vi "SetSystemDefinitionPropertyValue.vi"(8 "error in (no error)":errorcluster, 9 "value":string, 10 "property name":string, 11 "BaseNodeType in":refnum<k24>) -> (0 "error out":errorcluster, 3 "BaseNodeType out":refnum<k24>)   [LabVIEW 2015, in "VeriStandTestUtilities.lvlib"]
uses:
  VeriStandTestUtilities.lvlib
  NationalInstruments.VeriStand.SystemStorage
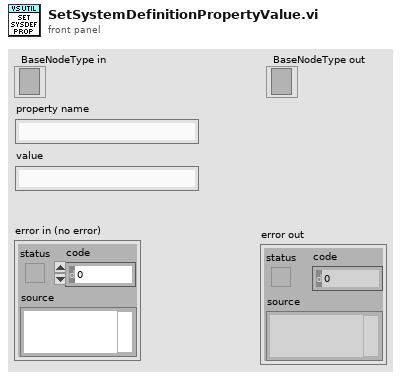
[diagram p1: front panel]
types:
  T1 = typedef "PropertyType.ctl" = enum16{"K_STRING", "K_BOOL", "K_I32", "K_U32", "K_DOUBLE", "K_U64", "K_VARIANT", "K_DEPENDENTFILE", "K_DEPENDENTNODE", "K_DATASOURCENODE", "K_U16", "K_DBLARR", "K_U32ARR", "K_I32ARR", "K_STRINGARR", "K_DICTIONARY", "K_DICTIONARYARR", "K_BINARYSTRING", "K_I16", "K_I64", "K_BOOLARR", "K_U64ARR", "K_U16ARR", "K_I64ARR", "K_I16ARR"}
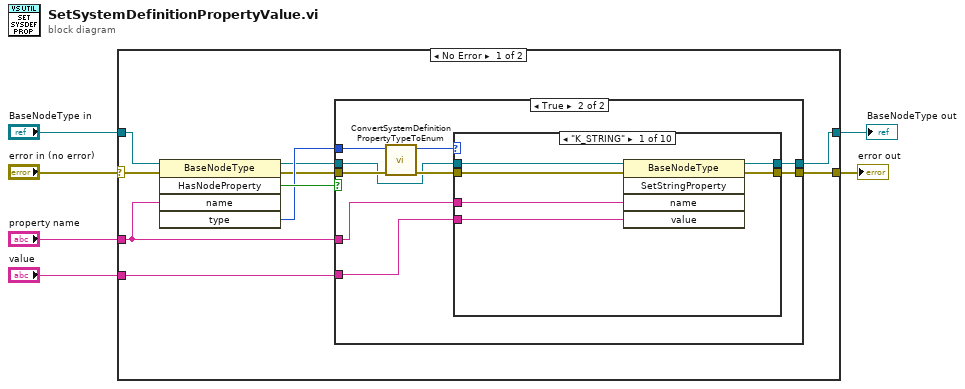
[diagram p0: block diagram]
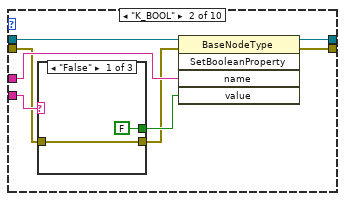
[diagram p3: hidden frame]
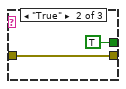
[diagram p4: hidden frame]
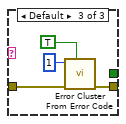
[diagram p5: hidden frame]
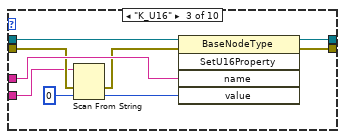
[diagram p6: hidden frame]
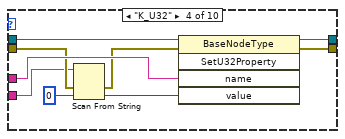
[diagram p7: hidden frame]
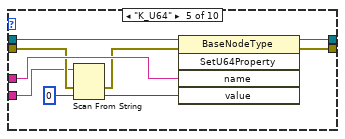
[diagram p8: hidden frame]
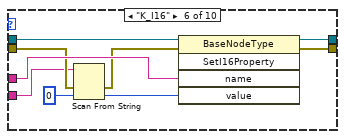
[diagram p9: hidden frame]
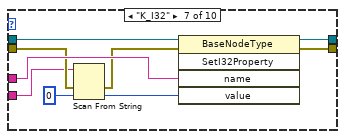
[diagram p10: hidden frame]
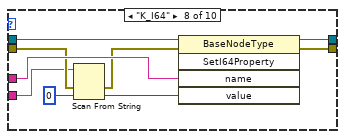
[diagram p11: hidden frame]
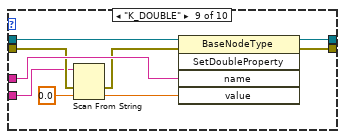
[diagram p12: hidden frame]
diagram:
  n1 = case shown="No Error" "error in (no error)" {
    selector: "error in (no error)" -> [w16 w116]
    tunnel: [w11 w116] -> w6
    tunnel: [w10 w115] -> w4
    tunnel: "BaseNodeType in" -> [w9 w115]
    tunnel: "property name" -> [w8 _]
    tunnel: "value" -> [w7 _]
    frame No Error {
      n2 = invoke class="BaseNodeType" method="HasNodeProperty"(reference=w9, error in=w16, "name"=w8) -> (reference out=w12:refnum<k24>, error out=w13:errorcluster, "HasNodeProperty"=w15:bool, "type"=w14:i32)  [unwired: 2 in, 1 out]
      n3 = case shown="True" w15 {
        tunnel: w14 -> [_ w27]
        tunnel: w13 -> [w17 w25]
        tunnel: w12 -> [w18 w23]
        tunnel: [w17 w22] -> w11
        tunnel: [w18 w21] -> w10
        tunnel: w8 -> [_ w20]
        tunnel: w7 -> [_ w19]
        frame False {
        }
        frame True {
          n4 = call "ConvertSystemDefinitionPropertyTypeToEnum.vi"("error in (no error)"=w25, "type"=w27) -> ("error out"=w24:errorcluster, "type"=w26:T1)  [unwired: 8 in]
          n5 = case shown="\"K_STRING\"" w26 {
            tunnel: w24 -> [w33 w35 w54 w63 w72 w81 w90 w99 w108 w113]
            tunnel: w23 -> [w32 w41 w58 w67 w76 w85 w94 w103 w112 w114]
            tunnel: [w31 w40 w57 w66 w75 w84 w93 w102 w111 w113] -> w22
            tunnel: [w30 w39 w56 w65 w74 w83 w92 w101 w110 w114] -> w21
            tunnel: w20 -> [w29 w38 w55 w64 w73 w82 w91 w100 w109 _]
            tunnel: w19 -> [w28 w37 w50 w59 w68 w77 w86 w95 w104 _]
            frame "K_STRING" {
              n6 = invoke class="BaseNodeType" method="SetStringProperty"(reference=w32, error in=w33, "name"=w29, "value"=w28) -> (reference out=w30:refnum<k24>, error out=w31:errorcluster)  [unwired: 1 in, 3 out]
            }
            frame "K_BOOL" {
              n7 = case shown="\"False\"" w37 {
                tunnel: [FALSE TRUE _] -> w36
                tunnel: w35 -> [w42 w44 w48]
                tunnel: [w42 w44 w49] -> w34
                frame "False" {
                }
                frame "True" {
                }
                frame Default {
                  n8 = call <vilib>:"Error Cluster From Error Code.vi"("show call chain? (False)"=TRUE, "error in (no error)"=w48, "error code (0)"=1) -> ("error out"=w49:errorcluster)  [unwired: 6 in]
                }
              }
              n9 = invoke class="BaseNodeType" method="SetBooleanProperty"(reference=w41, error in=w34, "name"=w38, "value"=w36) -> (reference out=w39:refnum<k24>, error out=w40:errorcluster)  [unwired: 1 in, 3 out]
            }
            frame "K_U16" {
              n10 = Scan From String(input string=w50, error in=w54, default 1=u16 0) -> (error out=w53:errorcluster, output 1=w51:u16)  [unwired: 2 in, 2 out]
              n11 = invoke class="BaseNodeType" method="SetU16Property"(reference=w58, error in=w53, "name"=w55, "value"=w51) -> (reference out=w56:refnum<k24>, error out=w57:errorcluster)  [unwired: 1 in, 3 out]
            }
            frame "K_U32" {
              n12 = Scan From String(input string=w59, error in=w63, default 1=u32 0) -> (error out=w62:errorcluster, output 1=w60:u32)  [unwired: 2 in, 2 out]
              n13 = invoke class="BaseNodeType" method="SetU32Property"(reference=w67, error in=w62, "name"=w64, "value"=w60) -> (reference out=w65:refnum<k24>, error out=w66:errorcluster)  [unwired: 1 in, 3 out]
            }
            frame "K_U64" {
              n14 = Scan From String(input string=w68, error in=w72, default 1=u64 0) -> (error out=w71:errorcluster, output 1=w69:u64)  [unwired: 2 in, 2 out]
              n15 = invoke class="BaseNodeType" method="SetU64Property"(reference=w76, error in=w71, "name"=w73, "value"=w69) -> (reference out=w74:refnum<k24>, error out=w75:errorcluster)  [unwired: 1 in, 3 out]
            }
            frame "K_I16" {
              n16 = Scan From String(input string=w77, error in=w81, default 1=i16 0) -> (error out=w80:errorcluster, output 1=w78:i16)  [unwired: 2 in, 2 out]
              n17 = invoke class="BaseNodeType" method="SetI16Property"(reference=w85, error in=w80, "name"=w82, "value"=w78) -> (reference out=w83:refnum<k24>, error out=w84:errorcluster)  [unwired: 1 in, 3 out]
            }
            frame "K_I32" {
              n18 = Scan From String(input string=w86, error in=w90, default 1=0) -> (error out=w89:errorcluster, output 1=w87:i32)  [unwired: 2 in, 2 out]
              n19 = invoke class="BaseNodeType" method="SetI32Property"(reference=w94, error in=w89, "name"=w91, "value"=w87) -> (reference out=w92:refnum<k24>, error out=w93:errorcluster)  [unwired: 1 in, 3 out]
            }
            frame "K_I64" {
              n20 = Scan From String(input string=w95, error in=w99, default 1=i64 0) -> (error out=w98:errorcluster, output 1=w96:i64)  [unwired: 2 in, 2 out]
              n21 = invoke class="BaseNodeType" method="SetI64Property"(reference=w103, error in=w98, "name"=w100, "value"=w96) -> (reference out=w101:refnum<k24>, error out=w102:errorcluster)  [unwired: 1 in, 3 out]
            }
            frame "K_DOUBLE" {
              n22 = Scan From String(input string=w104, error in=w108, default 1=0.0) -> (error out=w107:errorcluster, output 1=w105:dbl)  [unwired: 2 in, 2 out]
              n23 = invoke class="BaseNodeType" method="SetDoubleProperty"(reference=w112, error in=w107, "name"=w109, "value"=w105) -> (reference out=w110:refnum<k24>, error out=w111:errorcluster)  [unwired: 1 in, 3 out]
            }
            frame Default {
            }
          }
        }
      }
    }
    frame Error {
    }
  }
  "error out" <- w6
  "BaseNodeType out" <- w4
